vi "protoWindow.vi"() -> ()   [LabVIEW 2014]
uses:
  common/crest/LabVIEW/LV14/libcommon-crest.lvlib
panel:
  out "keys out":string
  out "values out":string
  out "parameters":string
  out "command":string
  out "element":string
  in  "Current Set [A]":dbl
  in  "set":bool
  in  "reset":bool
  in  "polaOpen":bool
  in  "polaPos":bool
  in  "polaNeg":bool
  out "fetch loop":i32
  out "index":i32
  in  "standby":bool
  in  "operational":bool
  in  "elementList":i32(listbox)
  in  "!CHAOS WAN url":string="192.168.150.91:8081"
  in  "enable window menu":bool
  in  "refreshConn":bool
  in  "set_to_saved":bool
  in  "local_load":bool
  in  "local_save":bool
  out "debug counter":i32
  # "ver. 1.0, build 20150320-1103"
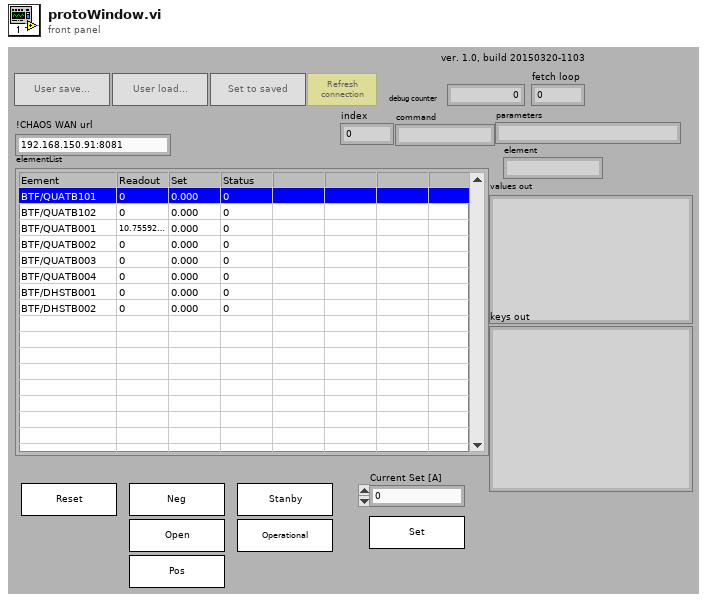
[diagram p1: front panel]
types:
  T1 = cluster{"numberOfElements":i32, "connectionHandle":u32, "statusFilter":i32, "mode":i32, "status":i32}
  T2 = cluster{"elementNames":string[], "staAddresses":u32[], "dynAddddresses":u32[], "classIDs":i32[], "VME/ETH":bool[]}
  T3 = typedef "LVRectTypeDef.ctl" = cluster{"Left":i16, "Top":i16, "Right":i16, "Bottom":i16}
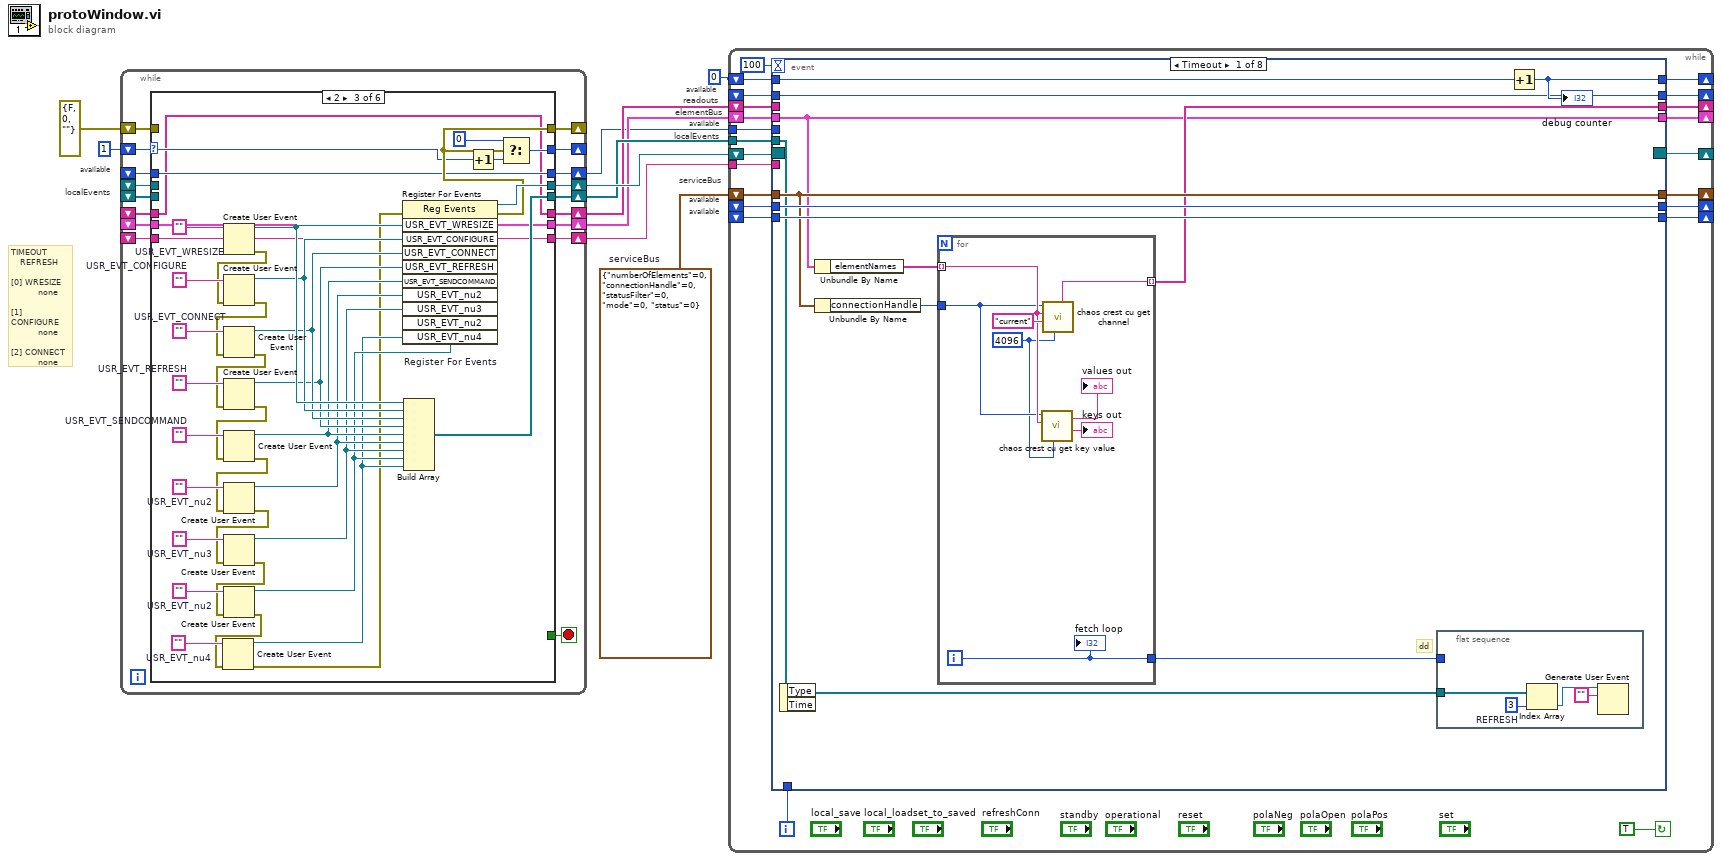
[diagram p0: block diagram]
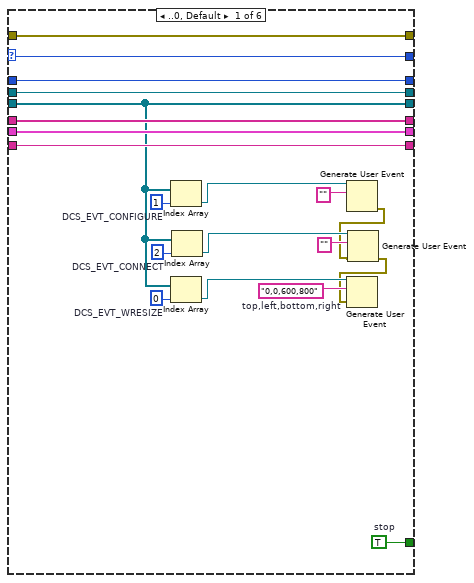
[diagram p2: hidden frame]
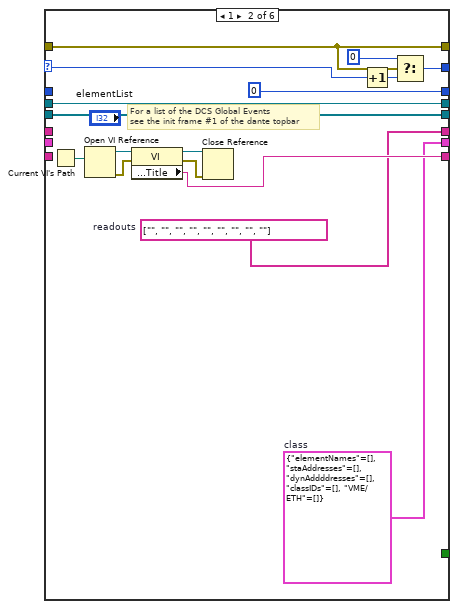
[diagram p3: hidden frame]
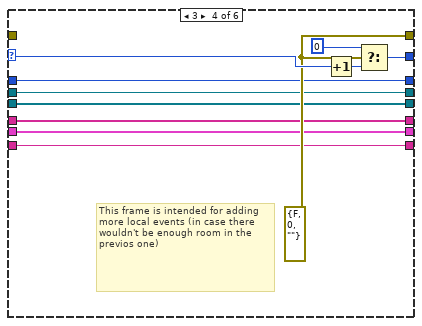
[diagram p4: hidden frame]
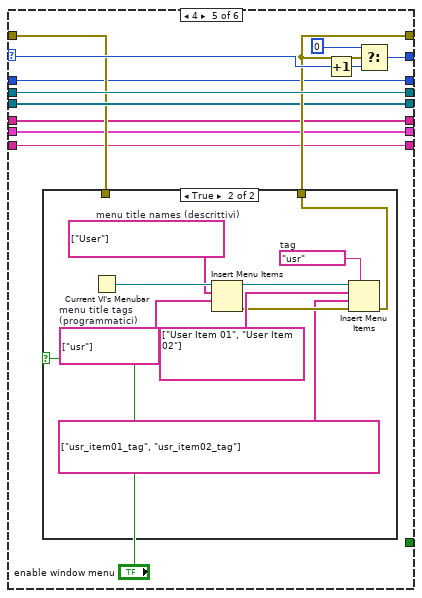
[diagram p5: hidden frame]
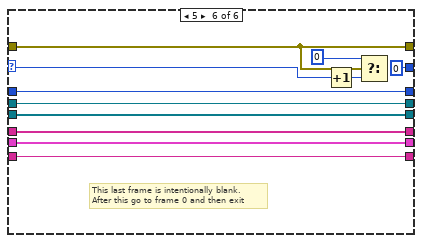
[diagram p7: hidden frame]
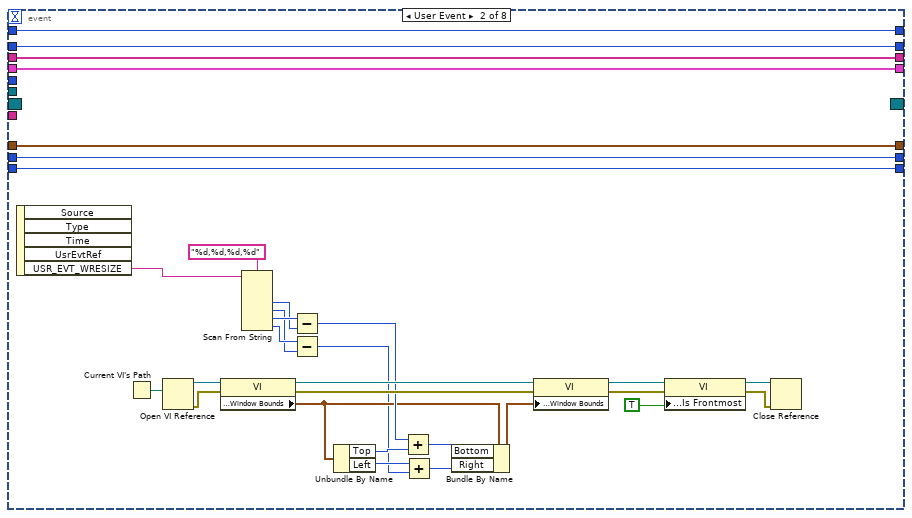
[diagram p8: hidden frame]
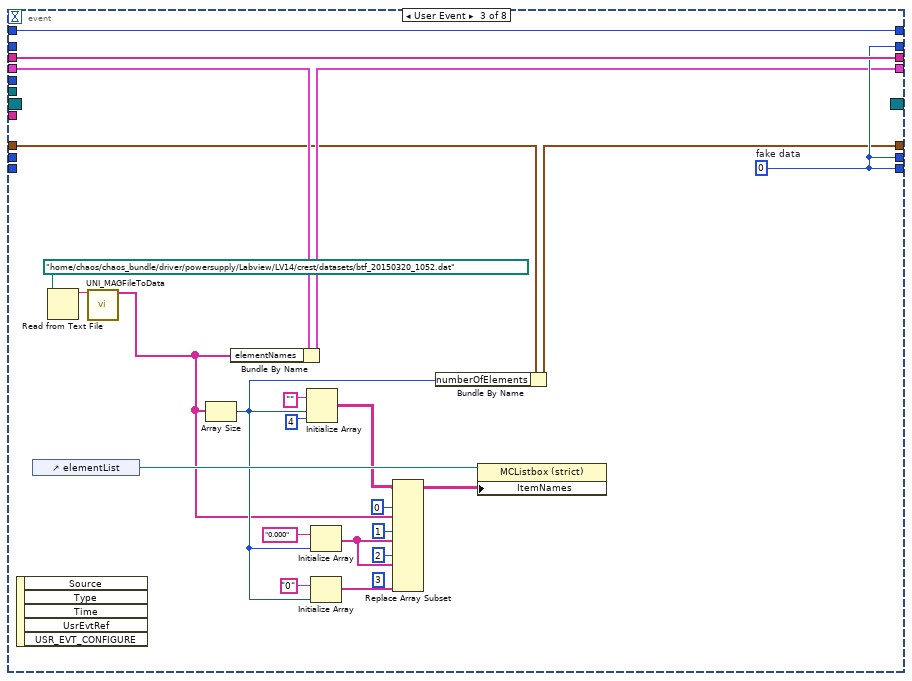
[diagram p9: hidden frame]
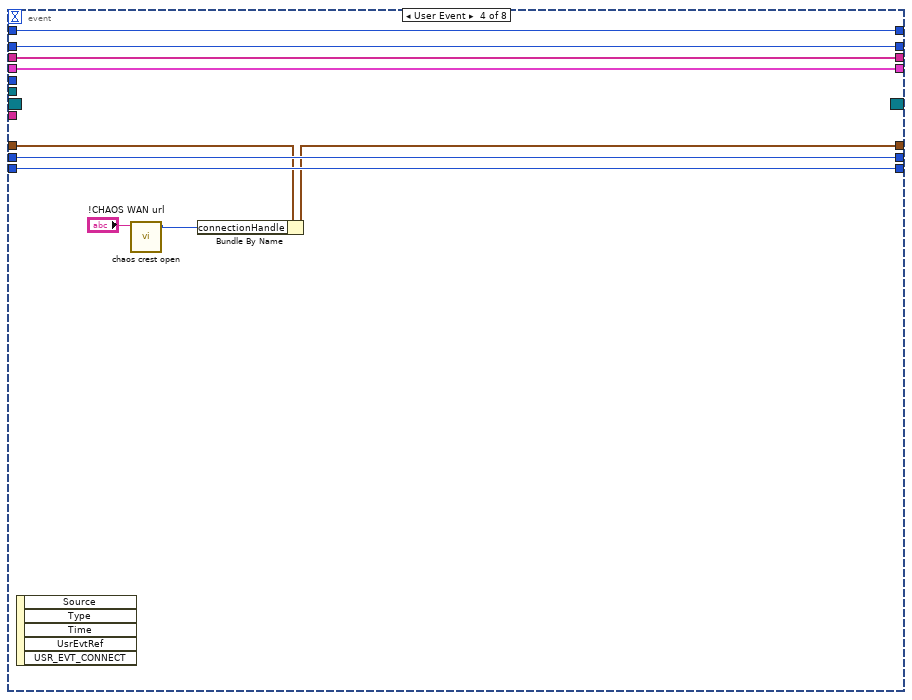
[diagram p10: hidden frame]
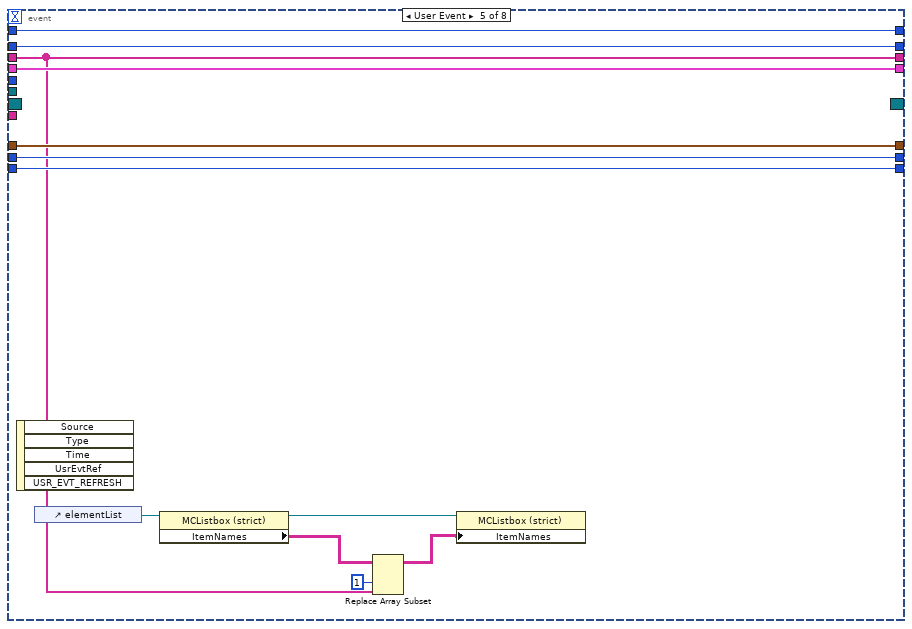
[diagram p11: hidden frame]
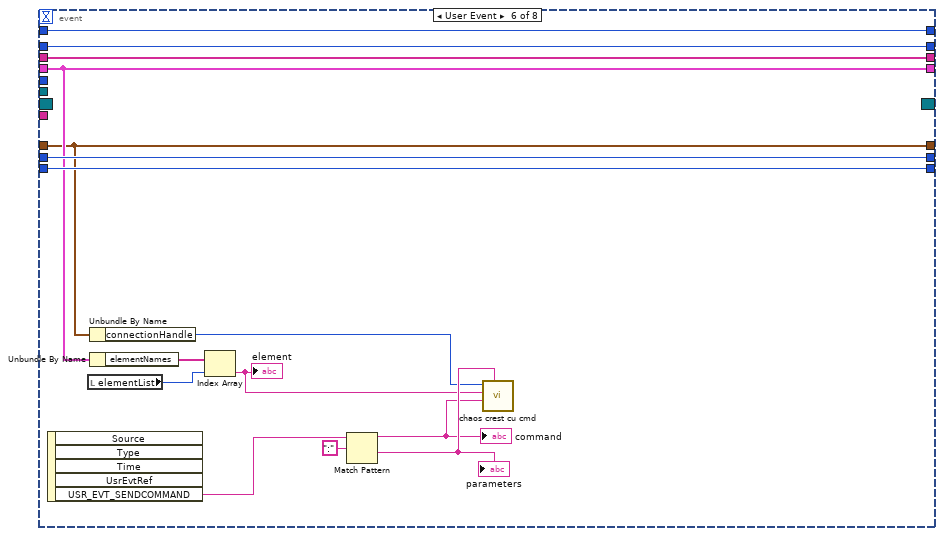
[diagram p12: hidden frame]
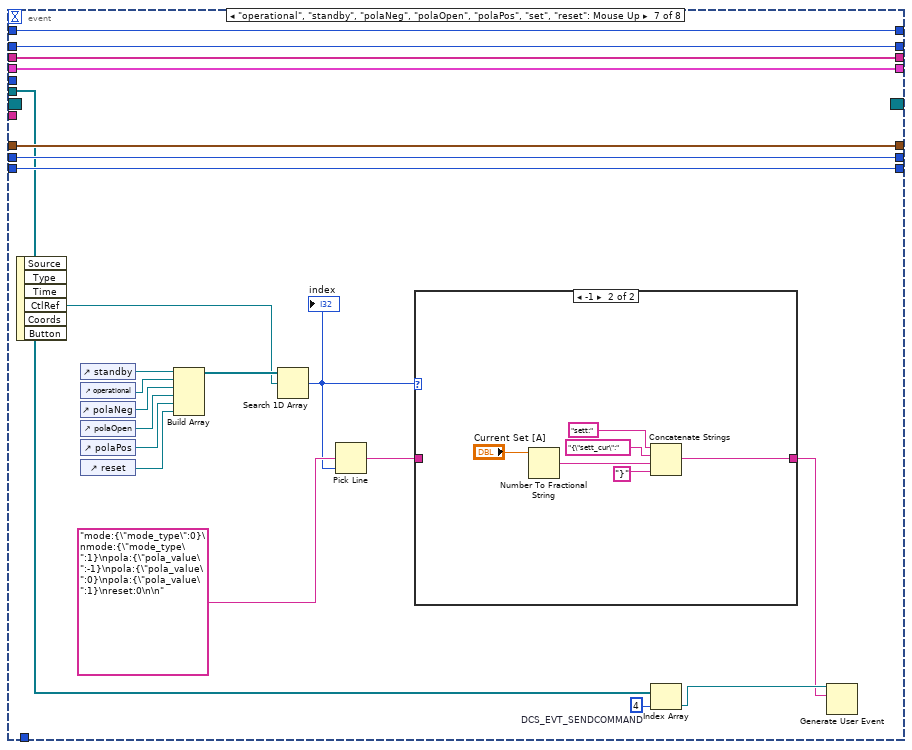
[diagram p13: hidden frame]
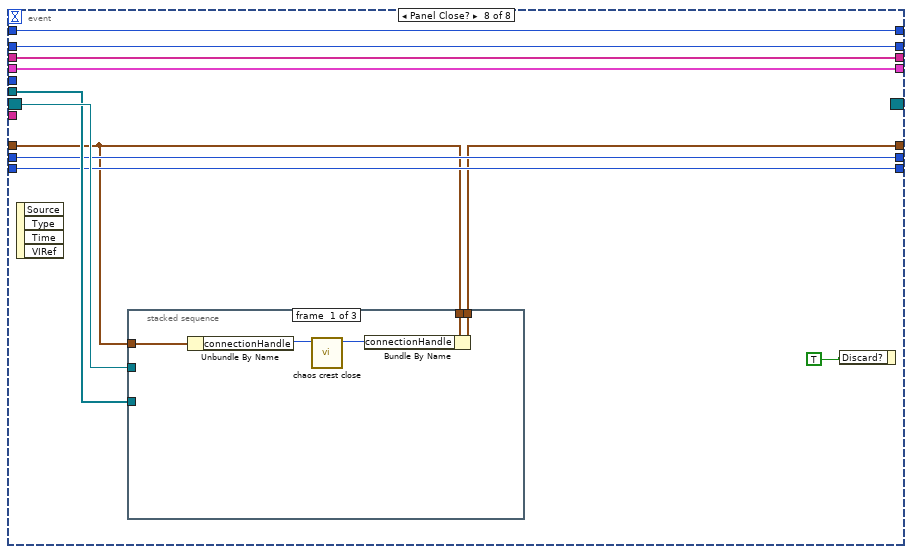
[diagram p15: hidden frame]
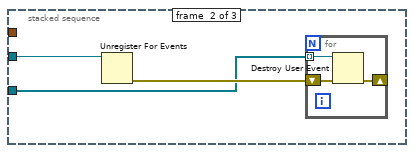
[diagram p16: hidden frame]
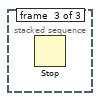
[diagram p17: hidden frame]
diagram:
  w4 = T1 {"numberOfElements"=0, "connectionHandle"=0, "statusFilter"=0, "mode"=0, "status"=0}  # serviceBus
  # "available"
  # "serviceBus"
  # "TIMEOUT\n   REFRESH\n\n[0] WRESIZE\n         none\n\n[1] CONFIGURE\n         none\n\n[2] CONNECT\n         none"
  # "localEvents"
  # "available"
  # "localEvents"
  # "available"
  # "readouts"
  # "elementBus"
  # "available"
  # "available"
  n1 = while {
    shift-right: [w21] -> _
    shift-left: 1 -> [w24]
    shift-right: [w26] -> w8
    shift-left: _ -> [w23]
    shift-right: [w27] -> w6
    shift-left: _ -> [w22]
    shift-right: [w20] -> _
    shift-left: errorcluster {"status"=FALSE, "code"=0, "source"=""} ("error out") -> [w19]
    shift-right: [w18] -> w7
    shift-left: _ -> [w17]
    shift-right: [w16] -> w5
    shift-left: _ -> [w15]
    shift-right: [w14] -> w3
    shift-left: _ -> [w13]
    shift-right: [w12] -> w2
    shift-left: _ -> [w11]
    stop <- w25 stop-if-true
    n2 = case shown="2" w24 {
      tunnel: [w45 w49 w65 w104 w116 w140] -> w27
      tunnel: [w46 w63 w97 w106 w125 w143] -> w26
      selector: w24 -> [w43 w51 w92 w109 w121 w144]
      tunnel: [w47 _ _ _ _ _] -> w25
      tunnel: w23 -> [w46 w63 _ w106 w125 w143]
      tunnel: w22 -> [w45 _ w65 w104 w116 w140]
      tunnel: [w43 w53 w94 w110 w124 0 ("t")] -> w21
      tunnel: [w44 w52 w93 w108 w120 w137] -> w20
      tunnel: w19 -> [w44 w52 _ _ w117 w137]
      tunnel: [w28 w62 w91 w105 w119 w142] -> w18
      tunnel: w17 -> [w28 w62 _ w105 w119 w142]
      tunnel: [w42 w50 w64 w103 w115 w139] -> w16
      tunnel: w15 -> [w42 _ w64 w103 w115 w139]
      tunnel: [w38 0 w74 w107 w114 w138] -> w14
      tunnel: w13 -> [w38 _ w74 w107 w114 w138]
      tunnel: [w33 w56 w66 w102 w113 w136] -> w12
      tunnel: w11 -> [w33 _ w66 w102 w113 w136]
      frame ..0, Default {
        w32 = 1  # DCS_EVT_CONFIGURE
        w35 = 2  # DCS_EVT_CONNECT
        w39 = "0,0,600,800"  # top,left,bottom,right
        w41 = 0  # DCS_EVT_WRESIZE
        w47 = TRUE  # stop
        n3 = Index Array(array=w28, index=w32) -> (element=w31:refnum<user-event>)
        n4 = Index Array(array=w28, index=w41) -> (element=w40:refnum<user-event>)
        n5 = Index Array(array=w28, index=w35) -> (element=w36:refnum<user-event>)
        n6 = Generate User Event(user event=w31, event data cluster="" ("event data")) -> (error out=w29:errorcluster)  [unwired: 2 in, 1 out]
        n7 = Generate User Event(user event=w36, event data cluster="" ("event data"), error in=w29) -> (error out=w34:errorcluster)  [unwired: 1 in, 1 out]
        n8 = Generate User Event(user event=w40, event data cluster=w39, error in=w34) -> ()  [unwired: 1 in, 2 out]
      }
      frame 1 {
        w50 = T2 {"elementNames"=[], "staAddresses"=[], "dynAddddresses"=[], "classIDs"=[], "VME/ETH"=[]}  # class
        w49 = string[] ["", "", "", "", "", "", "", "", ""]  # readouts
        # "For a list of the DCS Global Events\nsee the init frame #1 of the dante topbar"
        n9 = Current VI's Path() -> (path=w57:path)
        n10 = Open VI Reference(vi path=w57) -> (vi reference=w60:refnum<vi>, error out=w58:errorcluster)  [unwired: 5 in]
        n11 = property class="VI"(reference=w60, error in=w58) -> (reference out=w61:refnum<vi>, error out=w59:errorcluster, "Front Panel Window:Title"=w56:string)
        n12 = Close Reference(reference=w61, error in (no error)=w59) -> ()  [unwired: 1 out]
        n13 = Increment(x=w51) -> (x+1=w55:i32)
        n14 = Select(t=0, s=w52, f=w55) -> (s? t:f=w53:i32)
      }
      frame 2 {
        w70 = ""  # USR_EVT_nu4
        w73 = ""  # USR_EVT_nu2
        w80 = ""  # USR_EVT_nu3
        w83 = ""  # USR_EVT_nu2
        w86 = ""  # USR_EVT_SENDCOMMAND
        w88 = ""  # USR_EVT_REFRESH
        w90 = ""  # USR_EVT_CONNECT
        w98 = ""  # USR_EVT_CONFIGURE
        w101 = ""  # USR_EVT_WRESIZE
        n15 = Create User Event(user event datatype=w101) -> (user event=w100:refnum<user-event>, error out=w77:errorcluster)  [unwired: 1 in]
        n16 = Create User Event(user event datatype=w98, error in=w77) -> (user event=w99:refnum<user-event>, error out=w76:errorcluster)
        n17 = Create User Event(user event datatype=w90, error in=w76) -> (user event=w89:refnum<user-event>, error out=w75:errorcluster)
        n18 = Create User Event(user event datatype=w88, error in=w75) -> (user event=w87:refnum<user-event>, error out=w85:errorcluster)
        n19 = Create User Event(user event datatype=w86, error in=w85) -> (user event=w84:refnum<user-event>, error out=w82:errorcluster)
        n20 = Create User Event(user event datatype=w83, error in=w82) -> (user event=w81:refnum<user-event>, error out=w79:errorcluster)
        n21 = Create User Event(user event datatype=w80, error in=w79) -> (user event=w78:refnum<user-event>, error out=w72:errorcluster)
        n22 = Create User Event(user event datatype=w73, error in=w72) -> (user event=w71:refnum<user-event>, error out=w69:errorcluster)
        n23 = Create User Event(user event datatype=w70, error in=w69) -> (user event=w68:refnum<user-event>, error out=w67:errorcluster)
        n24 = register-events "Register For Events"(error in=w67, w100, w99, w89, w87, w84, w81, w78, w71, w68) -> (reference out=w97:refnum<event-registration>, error out=w93:errorcluster)  [unwired: 1 in]
        n25 = Build Array(w100, w99, w89, w87, w84, w81, w78, w71, w68) -> (w91:refnum<user-event>[])
        n26 = Increment(x=w92) -> (x+1=w96:i32)
        n27 = Select(t=0, s=w93, f=w96) -> (s? t:f=w94:i32)
      }
      frame 3 {
        w108 = errorcluster {"status"=FALSE, "code"=0, "source"=""} ("s")
        # "This frame is intended for adding more local events (in case there wouldn't be enough room in the previos one)"
        n28 = Increment(x=w109) -> (x+1=w112:i32)
        n29 = Select(t=0, s=w108, f=w112) -> (s? t:f=w110:i32)
      }
      frame 4 {
        n30 = case shown="True" "enable window menu" {
          tunnel: [w126 w127] -> w120
          tunnel: w117 -> [w126 _]
          frame False {
          }
          frame True {
            w134 = string[] ["User"]  # menu title names (descrittivi)
            w132 = "usr"  # tag
            w129 = string[] ["usr"]  # menu title tags (programmatici)
            n31 = Current VI's Menubar() -> (w135:refnum<k9>)
            n32 = Insert Menu Items(7:w129, 8:w134, 9:w135) -> (0:w130:errorcluster, 3:w131:refnum<k9>)  [unwired: 3 in, 1 out]
            n33 = Insert Menu Items(5:w132, 6:w130, 7:string[] ["usr_item01_tag", "usr_item02_tag"] ("item names"), 8:string[] ["User Item 01", "User Item 02"] ("item names"), 9:w131) -> (0:w127:errorcluster)  [unwired: 1 in, 2 out]
          }
        }
        n34 = Increment(x=w121) -> (x+1=w123:i32)
        n35 = Select(t=0, s=w120, f=w123) -> (s? t:f=w124:i32)
      }
      frame 5 {
        # "This last frame is intentionally blank.\nAfter this go to frame 0 and then exit"
        n36 = Increment(x=w144) -> (x+1=w146:i32)
        n37 = Select(t=0, s=w137, f=w146) -> ()  [unwired: 1 out]
      }
    }
  }
  n38 = while {
    shift-right: [w153] -> _
    shift-left: w6 -> [w154]
    shift-right: [w155] -> _
    shift-left: w5 -> [w156]
    shift-right: [w165] -> _
    shift-left: _ -> [w166]
    shift-right: [w167] -> _
    shift-left: _ -> [w164]
    shift-right: [w161] -> _
    shift-left: w8 -> [w163]
    tunnel: w7 -> [w162]
    shift-right: [w158] -> _
    shift-left: w4 -> [w159]
    tunnel: w3 -> [w157]
    tunnel: w2 -> [w152]
    shift-right: [w150] -> _
    shift-left: 0 ("debug counter") -> [w151]
    shift-right: [w148] -> _
    shift-left: _ -> [w149]
    i -> [w147]
    stop <- TRUE continue-if-true
    n39 = event shown="[0] Timeout" {
      selector: w163 -> [_ _ _ _ _ _ _ w322]
      dyn-events: [_ _ _ _ _ _ _ _] -> w161
      timeout: 100 -> [_ _ _ _ _ _ _ _]
      tunnel: [w176 w222 w244 w256 w267 w282 w304 w319] -> w167
      tunnel: w166 -> [w180 w223 _ w255 w268 w283 w305 w320]
      tunnel: [w180 w223 w244 w255 w268 w283 w305 w320] -> w165
      tunnel: w164 -> [w176 w222 _ w256 w267 w282 w304 w319]
      tunnel: w162 -> [w172 _ _ _ _ _ w288 w321]
      tunnel: w159 -> [w175 w217 w230 w249 w266 w271 w301 w314]
      tunnel: [w175 w217 w229 w248 w266 w271 w301 w313] -> w158
      tunnel: w157 -> [_ _ _ _ _ _ _ _]
      tunnel: w156 -> [w170 w220 w241 w250 w265 w278 w299 w317]
      tunnel: [w170 w220 w240 w250 w265 w278 w299 w317] -> w155
      tunnel: w154 -> [_ w221 w246 w252 w257 w281 w303 w318]
      tunnel: [w173 w221 w246 w252 w257 w281 w303 w318] -> w153
      tunnel: w152 -> [_ _ _ _ _ _ _ _]
      tunnel: w151 -> [w179 w216 w245 w254 w264 w280 w302 w316]
      tunnel: [w178 w216 w245 w254 w264 w280 w302 w316] -> w150
      tunnel: [w177 w215 w244 w253 w263 w279 w300 w315] -> w148
      tunnel: w149 -> [w177 w215 _ w253 w263 w279 w300 w315]
      tunnel: w147 -> [_ _ _ _ _ _ _ _]
      event Timeout {
        # "dd"
        n40 = event-data() -> ()  [unwired: 1 in, 2 out]
        n41 = Unbundle By Name(w170) -> ("elementNames"=w169:string[])
        n42 = Unbundle By Name(w175) -> ("connectionHandle"=w174:u32)
        n43 = for {
          tunnel: w174 -> [w188]
          tunnel: [w191] -> w173 mode=indexing
          tunnel: [w190] -> w171
          tunnel: w169 -> [w189] mode=indexing
          i -> [w190]
          w187 = 4096 ("maxsize")
          n44 = call "chaos crest cu get key value.vi"("maxsize"=w187, "cuname"=w189, "handleConnection"=w188) -> ("keys out"=→"keys out":string, "values out"=→"values out":string)  [unwired: 5 in, 2 out]
          n45 = call "chaos crest cu get channel.vi"("maxsize"=w187, "channame"="current", "cuname"=w189, "handleConnection"=w188) -> ("value out"=w191:string)  [unwired: 6 in, 1 out]
          "fetch loop" <- w190
        }
        n46 = flat-sequence {
          tunnel: w172 -> [w181]
          tunnel: w171 -> [_]
          frame #0 {
            w182 = 3  # REFRESH
            n47 = Index Array(array=w181, index=w182) -> (element=w183:refnum<user-event>)
            n48 = Generate User Event(user event=w183, event data cluster="" ("event data")) -> ()  [unwired: 2 in, 2 out]
          }
        }
        n49 = Increment(x=w179) -> (x+1=w178:i32)
        "debug counter" <- w178
      }
      event User Event {
        n50 = event-data() -> ("USR_EVT_WRESIZE"=w218:string)  [unwired: 1 in, 4 out]
        n51 = Current VI's Path() -> (path=w209:path)
        n52 = Open VI Reference(vi path=w209) -> (vi reference=w208:refnum<vi>, error out=w207:errorcluster)  [unwired: 5 in]
        n53 = property class="VI"(reference=w208, error in=w207) -> (reference out=w205:refnum<vi>, error out=w206:errorcluster, "Front Panel Window:Window Bounds"=w201:T3)
        n54 = Scan From String(format string="%d,%d,%d,%d", input string=w218) -> (output 1=w203:i32, output 2=w196:i32, output 3=w204:i32, output 4=w197:i32)  [unwired: 6 in, 3 out]
        n55 = Subtract(x=w204, y=w203) -> (x-y=w202:i32)
        n56 = Subtract(x=w197, y=w196) -> (x-y=w194:i32)
        n57 = Unbundle By Name(w201) -> ("Top"=w199:i16, "Left"=w195:i16)
        n58 = Add(x=w202, y=w199) -> (x+y=w198:i32)
        n59 = Add(x=w195, y=w194) -> (x+y=w193:i32)
        n60 = Bundle By Name(cluster=w201, "Bottom"=w198, "Right"=w193) -> (w200:T3)
        n61 = property class="VI"(reference=w205, error in=w206, "Front Panel Window:Window Bounds"=w200) -> (reference out=w210:refnum<vi>, error out=w211:errorcluster)
        n62 = property class="VI"(reference=w210, error in=w211, "Front Panel Window:Is Frontmost"=TRUE) -> (reference out=w213:refnum<vi>, error out=w214:errorcluster)
        n63 = Close Reference(reference=w213, error in (no error)=w214) -> ()  [unwired: 1 out]
      }
      event User Event {
        (unwired) 3 ("disabled index (col)")
        w244 = 0  # fake data
        n64 = event-data() -> ()  [unwired: 1 in, 5 out]
        n65 = control-ref of="elementList"() -> (w237:refnum<vi>)
        n66 = Read from Text File(file (use dialog)=path "/home/chaos/chaos_bundle/driver/powersupply/Labview/LV14/crest/datasets/btf_20150320_1052.dat" ("new file path (Not A Path if cancelled)")) -> (text=w243:string)  [unwired: 3 in, 3 out]
        n67 = call "UNI_MAGFileToData.vi"("spreadsheetData"=w243) -> ("names"=w224:string[])  [unwired: 6 in, 8 out]
        n68 = Array Size(array=w224) -> (size(s)=w226:i32)
        n69 = Bundle By Name(cluster=w241, "elementNames"=w224) -> (w240:T2)
        n70 = Initialize Array("" ("event data"), w226, 4 ("dimension size")) -> (w235:string[][])
        n71 = Initialize Array("0.000" ("event data"), w226) -> (w231:string[])
        n72 = Initialize Array("0" ("event data"), w226) -> (w225:string[])
        n73 = Replace Array Subset(array=w235, new element #1=w224, index (col) #1=0 ("disabled index (col)"), new element #2=w231, index (col) #2=1 ("disabled index (col)"), new element #3=w231, index (col) #3=2 ("disabled index (col)"), new element #4=w225) -> (w238:string[][])  [unwired: 5 in]
        n74 = Bundle By Name(cluster=w230, "numberOfElements"=w226) -> (w229:T1)
        n75 = property class="MCListbox (strict)"(reference=w237, "ItemNames"=w238) -> ()  [unwired: 1 in, 2 out]
      }
      event User Event {
        n76 = event-data() -> ()  [unwired: 1 in, 5 out]
        n77 = call "chaos crest open.vi"("chaoswanurl"="!CHAOS WAN url") -> ("handleConnection"=w247:u32)  [unwired: 10 in]
        n78 = Bundle By Name(cluster=w249, "connectionHandle"=w247) -> (w248:T1)
      }
      event User Event {
        n79 = event-data() -> ()  [unwired: 1 in, 5 out]
        n80 = control-ref of="elementList"() -> (w261:refnum<vi>)
        n81 = property class="MCListbox (strict)"(reference=w261) -> (reference out=w260:refnum<vi>, "ItemNames"=w259:string[][])  [unwired: 1 in, 1 out]
        n82 = Replace Array Subset(array=w259, new element=w257, index (col)=1 ("disabled index (col)")) -> (w258:string[][])  [unwired: 1 in]
        n83 = property class="MCListbox (strict)"(reference=w260, "ItemNames"=w258) -> ()  [unwired: 1 in, 2 out]
      }
      event User Event {
        n84 = event-data() -> ("USR_EVT_SENDCOMMAND"=w274:string)  [unwired: 1 in, 4 out]
        n85 = local read "elementList"() -> (w276:i32)
        n86 = Unbundle By Name(w271) -> ("connectionHandle"=w270:u32)
        n87 = Unbundle By Name(w278) -> ("elementNames"=w277:string[])
        n88 = Index Array(array=w277, index=w276) -> (element=w269:string)
        "element" <- w269
        n89 = Match Pattern(string=w274, regular expression=":") -> (before substring=w272:string, after substring=w273:string)  [unwired: 1 in, 2 out]
        "command" <- w272
        "parameters" <- w273
        n90 = call "chaos crest cu cmd.vi"("args"=w273, "cmd"=w272, "cuname"=w269, "handleConnection"=w270) -> ()  [unwired: 7 in, 1 out]
      }
      event "operational", "standby", "polaNeg", "polaOpen", "polaPos", "set", "reset": Mouse Up {
        w290 = 4  # DCS_EVT_SENDCOMMAND
        n91 = event-data() -> ("CtlRef"=w297:refnum<vi>)  [unwired: 1 in, 5 out]
        n92 = control-ref of="standby"() -> (w295:refnum<vi>)
        n93 = control-ref of="operational"() -> (w294:refnum<vi>)
        n94 = control-ref of="polaNeg"() -> (w293:refnum<vi>)
        n95 = control-ref of="polaOpen"() -> (w292:refnum<vi>)
        n96 = control-ref of="polaPos"() -> (w291:refnum<vi>)
        n97 = control-ref of="reset"() -> (w284:refnum<vi>)
        n98 = Build Array(w295, w294, w293, w292, w291, w284) -> (w298:refnum<vi>[])
        n99 = Search 1D Array(1D array=w298, element=w297) -> (index of element=w285:i32)  [unwired: 1 in]
        "index" <- w285
        n100 = Pick Line(multi-line string="mode:{\"mode_type\":0}\nmode:{\"mode_type\":1}\npola:{\"pola_value\":-1}\npola:{\"pola_value\":0}\npola:{\"pola_value\":1}\nreset:0\n\n", line index=w285) -> (output string=w287:string)  [unwired: 1 in]
        n101 = case shown="-1" w285 {
          tunnel: w287 -> [w306 _]
          tunnel: [w306 w308] -> w286
          frame Default {
          }
          frame -1 {
            n102 = Number To Fractional String(number="Current Set [A]") -> (F-format string=w310:string)  [unwired: 3 in]
            n103 = Concatenate Strings("sett:" ("cmd"), "{\"sett_cur\":", w310, "}" ("string")) -> (w308:string)
          }
        }
        n104 = Index Array(array=w288, index=w290) -> (element=w289:refnum<user-event>)
        n105 = Generate User Event(user event=w289, event data cluster=w286) -> ()  [unwired: 2 in, 2 out]
      }
      event Panel Close? {
        n106 = event-data() -> ()  [unwired: 1 in, 4 out]
        n107 = stacked-sequence {
          tunnel: w322 -> [_ w330 _]
          tunnel: w321 -> [_ w329 _]
          tunnel: w314 -> [w327 _ _]
          tunnel: w314 -> [w326 _ _]
          tunnel: [w325 _ _] -> w313
          frame #0 {
            n108 = Unbundle By Name(w327) -> ("connectionHandle"=w328:u32)
            n109 = call "chaos crest close.vi"("connectionHandle"=w328) -> ("connectionHandle out"=w324:u32)  [unwired: 9 in, 1 out]
            n110 = Bundle By Name(cluster=w326, "connectionHandle"=w324) -> (w325:T1)
          }
          frame #1 {
            n111 = Unregister For Events(event registration refnum=w330) -> (error out=w331:errorcluster)  [unwired: 1 in]
            n112 = for {
              tunnel: w329 -> [w334] mode=indexing
              shift-right: [w332] -> _
              shift-left: w331 -> [w333]
              n113 = Destroy User Event(user event=w334, error in=w333) -> (error out=w332:errorcluster)
            }
          }
          frame #2 {
            n114 = Stop() -> ()  [unwired: 1 in]
          }
        }
        n115 = event-data("Discard?"=TRUE) -> ()  [unwired: 1 in, 1 out]
      }
    }
  }
